vi "Anritsu VNA Read Sweep Time.vi"(6 "Channel":i8=1 min=1 max=99 step=1, 7 "Anritsu VNA":T1, 8 "error in (no error)":errorcluster, 11 "VISA Resource Name":refnum<visa-resource-name>) -> (0 "error out":errorcluster, 2 "Sweep Time, s":dbl=3000.0, 3 "dup VISA Resource Name":refnum<visa-resource-name>)   [LabVIEW 2011]
doc: "This Vi for the HP8753B Network Analyzer is used to set averaging, smoothing, and the IF bandwidth."
uses:
  TypeDefs/Anritsu VNA Instrument Info.ctl
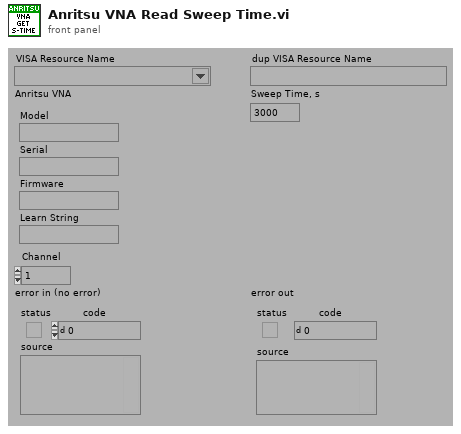
[diagram p1: front panel]
types:
  T1 = typedef "Anritsu VNA Instrument Info.ctl" = cluster{"Model":string, "Serial":string, "Firmware":string, "Learn String":string}
  T2 = typedef "Anritsu VNA Model.ctl" = enum16{"Not Supported", "37XXXX", "MS20XXX", "MS462XX", "MS464XX"}
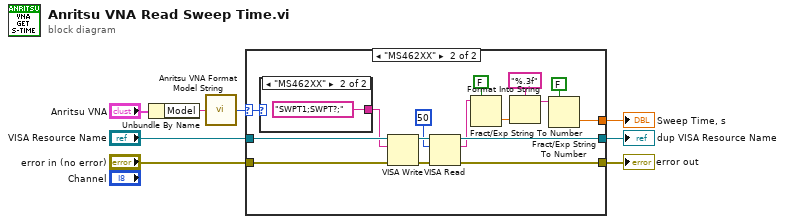
[diagram p0: block diagram]
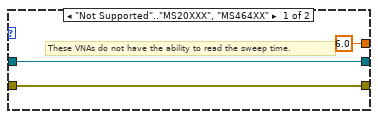
[diagram p2: hidden frame]
diagram:
  n1 = Unbundle By Name("Anritsu VNA") -> ("Model"=w2:string)
  n2 = call "Anritsu VNA Format Model String.vi"("Model"=w2) -> ("Model"=w1:T2)
  n3 = case shown="\"MS462XX\"" w1 {
    selector: w1 -> [_ w12]
    tunnel: "VISA Resource Name" -> [w11 w27]
    tunnel: "error in (no error)" -> [w10 w26]
    tunnel: [w11 w24] -> w6
    tunnel: [w10 w20] -> w5
    tunnel: [6.0 w14] -> w4
    frame "Not Supported".."MS20XXX", "MS464XX" {
      # "These VNAs do not have the ability to read the sweep time."
    }
    frame "MS462XX" {
      n4 = case shown="\"MS462XX\"" w12 {
        tunnel: [_ "SWPT1;SWPT?;"] -> w13
        frame "Not Supported".."MS20XXX", "MS464XX" {
        }
        frame "MS462XX" {
        }
      }
      n5 = VISA Write(VISA resource name=w27, write buffer=w13, error in (no error)=w26) -> (VISA resource name out=w25:refnum<visa-resource-name>, error out=w21:errorcluster)  [unwired: 1 out]
      n6 = VISA Read(VISA resource name=w25, byte count=u32 50, error in (no error)=w21) -> (VISA resource name out=w24:refnum<visa-resource-name>, read buffer=w16:string, error out=w20:errorcluster)  [unwired: 1 out]
      n7 = Fract/Exp String To Number(use system decimal point (T)=FALSE, string=w16) -> (number=w19:dbl)  [unwired: 3 out]
      n8 = Format Into String(format string="%.3f", w19) -> (resulting string=w18:string)  [unwired: 2 in, 1 out]
      n9 = Fract/Exp String To Number(use system decimal point (T)=FALSE, string=w18) -> (number=w14:dbl)  [unwired: 3 out]
    }
  }
  "error out" <- w5
  "dup VISA Resource Name" <- w6
  "Sweep Time, s" <- w4
